vi "Generate Waterfall Plots.vi"(8 "# Plots (10)":i32=10, 9 "Waterfall Age (30 sec)":dbl=30.0 format="%#_13g", 10 "Data Timestamp":timestamp, 11 "00-02-9234 Power Spectras":cluster{"f0":dbl, "df":dbl, "magnitude":dbl[]}[](array[cluster])) -> (1 "Fan Waterfall":T1, 2 "Gearbox Waterfwall":T1, 3 "Power Section RMS Waterfall":T1)   [LabVIEW 2014, in "Testing UI 3.lvlib"]
uses:
  Testing UI 3.lvlib
  <vilib>/Analysis/baseanly.llb/Histogram.vi
  <vilib>/Analysis/baseanly.llb/Mean.vi
  <vilib>/Analysis/baseanly.llb/Mean (DBL).vi
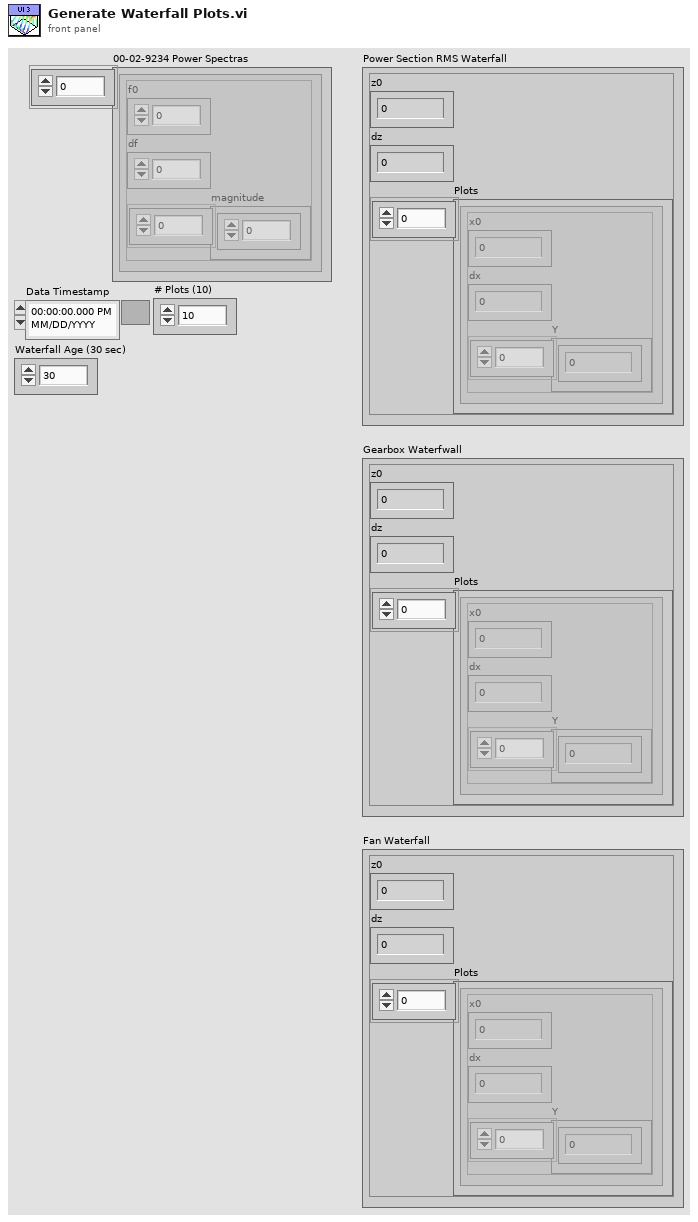
[diagram p1: front panel]
types:
  T1 = cluster{"z0":dbl, "dz":dbl, "Plots":cluster{"x0":dbl, "dx":dbl, "Y":dbl[]}[]}
  T2 = cluster{"power spectrum [dB EU]":cluster{"f0":dbl, "df":dbl, "magnitude":dbl[]}, "Data Timestamp":dbl}[]
  T3 = cluster{"power spectrum [dB EU]":cluster{"f0":dbl, "df":dbl, "magnitude":dbl[]}, "Data Timestamp":dbl}
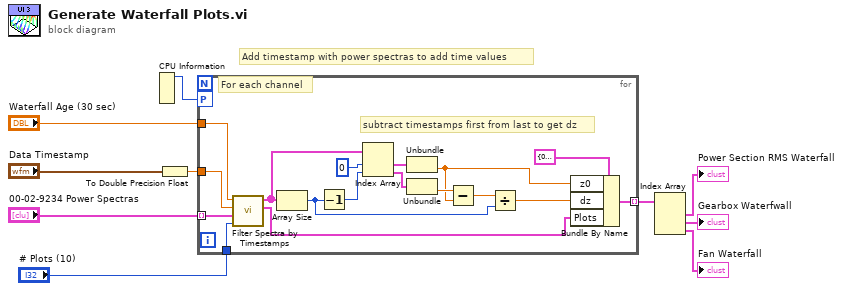
[diagram p0: block diagram]
diagram:
  # "Add timestamp with power spectras to add time values"
  n1 = CPU Information() -> (4:w2:i32)  [unwired: 3 out]
  n2 = To Double Precision Float(number="Data Timestamp") -> (double precision float=w8:dbl)
  n3 = for {
    tunnel: "00-02-9234 Power Spectras" -> [w27] mode=indexing
    tunnel: w8 -> [w25]
    tunnel: "Waterfall Age (30 sec)" -> [w26]
    tunnel: [w13] -> w6 mode=indexing
    workers-P: w2 -> [_]
    tunnel: "# Plots (10)" -> [w11]
    # "subtract timestamps first from last to get dz"
    # "For each channel"
    n4 = call "Filter Spectra by Timestamps.vi"("# Plots (10)"=w11, "Single Spectrum"=w27, "Data Timestamp"=w25, "Waterfall Age"=w26) -> ("Spectra to Plot"=w22:cluster{"f0":dbl, "df":dbl, "magnitude":dbl[]}[], "Spectra Plot with Timestamp"=w21:T2)  [unwired: 6 in]
    n5 = Array Size(array=w21) -> (size(s)=w14:i32)
    n6 = Decrement(x=w14) -> (x-1=w19:i32)
    n7 = Index Array(array=w21, index #1=0 ("index"), index #2=w19) -> (element #1=w24:T3, element #2=w18:T3)
    n8 = Unbundle(w24) -> ("Data Timestamp"=w16:dbl)  [unwired: 1 out]
    n9 = Unbundle(w18) -> ("Data Timestamp"=w17:dbl)  [unwired: 1 out]
    n10 = Subtract(x=w17, y=w16) -> (x-y=w15:dbl)
    n11 = Divide(x=w15, y=w14) -> (x/y=w12:dbl)
    n12 = Bundle By Name(cluster=T1 {"z0"=0.0, "dz"=0.0, "Plots"=[]} ("Fan Waterfall"), "z0"=w16, "dz"=w12, "Plots"=w22) -> (w13:T1)
  }
  n13 = Index Array(array=w6) -> (element #1=→"Power Section RMS Waterfall":T1, element #2=→"Gearbox Waterfwall":T1, element #3=→"Fan Waterfall":T1)  [unwired: 3 in]
